vi "Close.vi"(0 "UART Driver in":refnum<class "UART Driver.lvclass">, 5 "Force Reset UART? (T)":bool=TRUE, 11 "error in":errorcluster) -> (15 "error out":errorcluster)   [LabVIEW 2012, in "UART_Host_Driver.lvlib" / "UART Driver.lvclass"]
doc: "Close the UART Session.\n\nMust call UART Initialize.vi, prior to calling UART Close.vi."
uses:
  UART Driver.lvclass
  Typedefs/FPGA VI Reference.ctl
  UART Driver.lvclass/UART Driver.ctl
  <vilib>/FPGAPlugInAG/Dynamic/niLvFpga_Close_Dynamic.vi
  <vilib>/rvi/interface/nirviCloseFPGA/nirviCloseFPGA.xnode
  UART_Host_Driver.lvlib
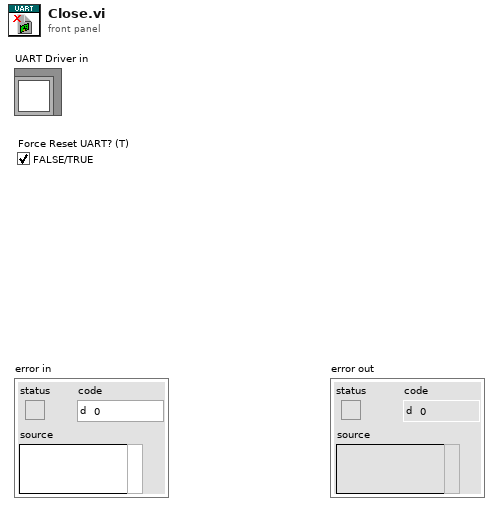
[diagram p1: front panel]
types:
  T1 = typedef "UART_Host_Driver.lvlib/FPGA VI Reference.ctl" = refnum<k20>
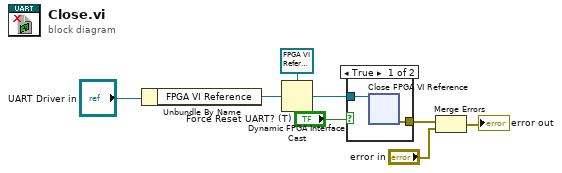
[diagram p0: block diagram]
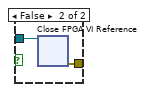
[diagram p2: hidden frame]
diagram:
  n1 = Unbundle By Name("UART Driver in") -> ("FPGA VI Reference"=w6:refnum<k20>)
  n2 = Dynamic FPGA Interface Cast(Session In=T1 refnum ("FPGA VI Reference"), Type=w6) -> (Session Out=w5:T1)
  n3 = case shown="True" "Force Reset UART? (T)" {
    tunnel: w5 -> [w10 w12]
    tunnel: [w9 w11] -> w4
    frame True {
      n4 = xnode "Close FPGA VI Reference"("FPGA VI Reference In"=w10) -> ("error out"=w9:errorcluster)  [unwired: 1 in]
    }
    frame False {
      n5 = xnode "Close FPGA VI Reference"("FPGA VI Reference In"=w12) -> ("error out"=w11:errorcluster)  [unwired: 1 in]
    }
  }
  n6 = Merge Errors(w4, "error in") -> (→"error out":errorcluster)
